vi "niDTS Comm String Set Parameters EXE.vi"(0 "Comm String Handle":T2, 5 "EXE Path":path, 7 "Port Parameters EXE":T1={"Timeout (s)"=5.0}, 11 "error in (no error)":errorcluster) -> (4 "Comm String Handle Out":T2, 15 "error out":errorcluster)   [LabVIEW 2014, in "niDTS CommLib.lvlib"]
doc: "This sends the Command concatenated with the Args over the String Interface.\n\nInputs:\n* Command (Required): This is the command to be sent.\n* Args (Optional): Any arguments to be concatenated with the command.\n\nOutputs:\n* Response: Any data returned from the interface. Note that no data wil be returned if the flag Read Enabled is set to FALSE."
uses:
  niDTS CommLib.lvlib
  Includes/niDTS Comm String INC Handle.ctl
  Objects/String_class/niDTS Comm String.lvclass
  Includes/niDTS Comm INC EXE Port Parameters.ctl
  Includes/niDTS Comm EXE INC Handle.ctl
  Objects/EXE_class/niDTS Comm EXE.lvclass
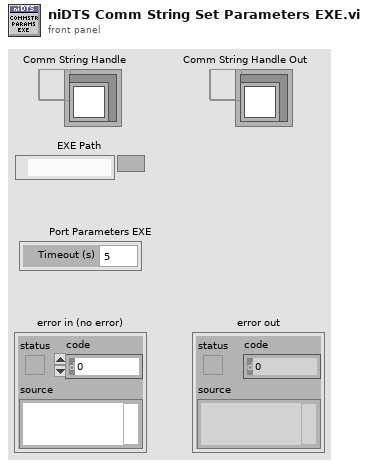
[diagram p1: front panel]
types:
  T1 = typedef "niDTS CommLib.lvlib/niDTS Comm INC EXE Port Parameters.ctl" = cluster{"Timeout (s)":dbl}
  T2 = typedef "niDTS CommLib.lvlib/niDTS Comm String INC Handle.ctl" = refnum<data-value>
  T3 = typedef "niDTS CommLib.lvlib/niDTS Comm EXE INC Handle.ctl" = refnum<data-value>
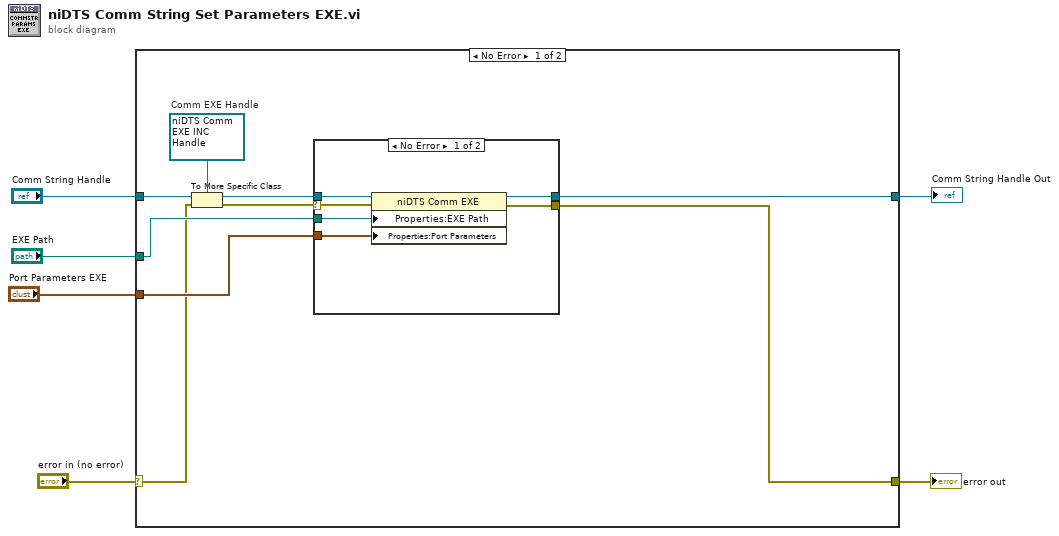
[diagram p0: block diagram]
diagram:
  n1 = case shown="No Error" "error in (no error)" {
    selector: "error in (no error)" -> [w8 w25]
    tunnel: [w7 w25] -> w6
    tunnel: "Comm String Handle" -> [w15 w24]
    tunnel: [w9 w24] -> w4
    tunnel: "EXE Path" -> [w11 _]
    tunnel: "Port Parameters EXE" -> [w10 _]
    frame No Error {
      w14 = T3 refnum  # Comm EXE Handle
      n2 = To More Specific Class(target class=w14, reference=w15, error in=w8) -> (specific class reference=w12:T3, error out=w13:errorcluster)
      n3 = case shown="No Error" w13 {
        selector: w13 -> [w20 w22]
        tunnel: w12 -> [w21 w23]
        tunnel: w11 -> [w19 _]
        tunnel: w10 -> [w18 _]
        tunnel: [w17 w23] -> w9
        tunnel: [w16 w22] -> w7
        frame No Error {
          n4 = property class="niDTS Comm EXE"(reference=w21, error in=w20, "Properties:EXE Path"=w19, "Properties:Port Parameters"=w18) -> (reference out=w17:T3, error out=w16:errorcluster)
        }
        frame Error {
        }
      }
    }
    frame Error {
    }
  }
  "error out" <- w6
  "Comm String Handle Out" <- w4
